vi "Sort_Destinations.vi"(8 "error in (no error)":errorcluster, 11 "Installer in":refnum<class "Installer.lvclass">) -> (0 "error out":errorcluster, 3 "Installer out":refnum<class "Installer.lvclass">)   [LabVIEW 2020, in "Installer.lvclass"]
uses:
  <vilib>/AppBuilder/IB_Classes/Installer/Installer.lvclass
  <vilib>/AppBuilder/IB_Classes/Installer/Installer.lvclass/Installer.ctl
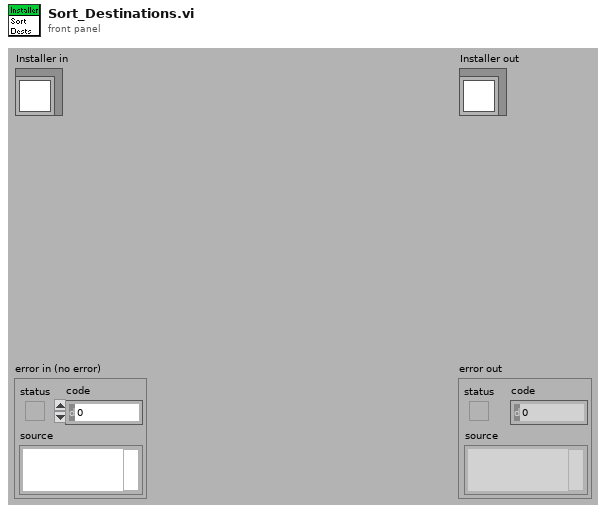
[diagram p1: front panel]
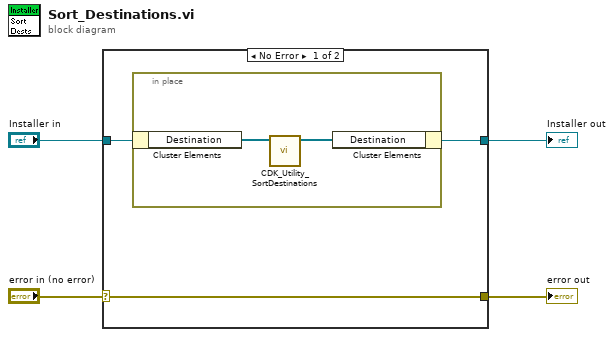
[diagram p0: block diagram]
diagram:
  n1 = case shown="No Error" "error in (no error)" {
    selector: "error in (no error)" -> [w7 w11]
    tunnel: [w7 w11] -> w3
    tunnel: [w5 w10] -> w1
    tunnel: "Installer in" -> [w6 w10]
    frame No Error {
      n2 = in-place {
        n3 = in-place-cluster #1(w6) -> ("Destination"=w8:refnum<class "IB_Destination.lvclass">[])
        n4 = call <resource>:"CDK_Utility_SortDestinations.vi"("dests"=w8) -> ("sorted dests"=w9:refnum<class "IB_Destination.lvclass">[])  [unwired: 10 out]
        n5 = in-place-cluster #1("Destination"=w9) -> (w5:refnum<class "Installer.lvclass">)
      }
    }
    frame Error {
    }
  }
  "error out" <- w3
  "Installer out" <- w1
